vi "ReferenceChannelsToSave.vi"(8 "error in":errorcluster) -> (0 "error out":errorcluster, 1 "Item Names":string[](array[string]), 2 "Value":i32[](array[numeric]), 3 "referenceListBox":refnum<vi>)   [LabVIEW 2016]
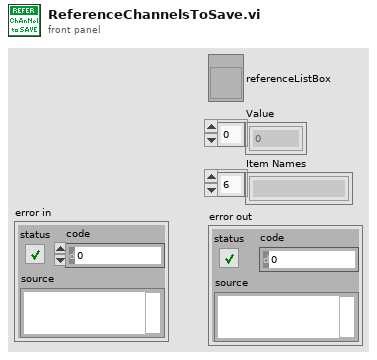
[diagram p1: front panel]
types:
  T1 = enum32{"Invalid", "Standard", "Closed", "Hidden", "Minimized", "Maximized"}
  T2 = enum32{"Bad", "Idle", "Run top level", "Running"}
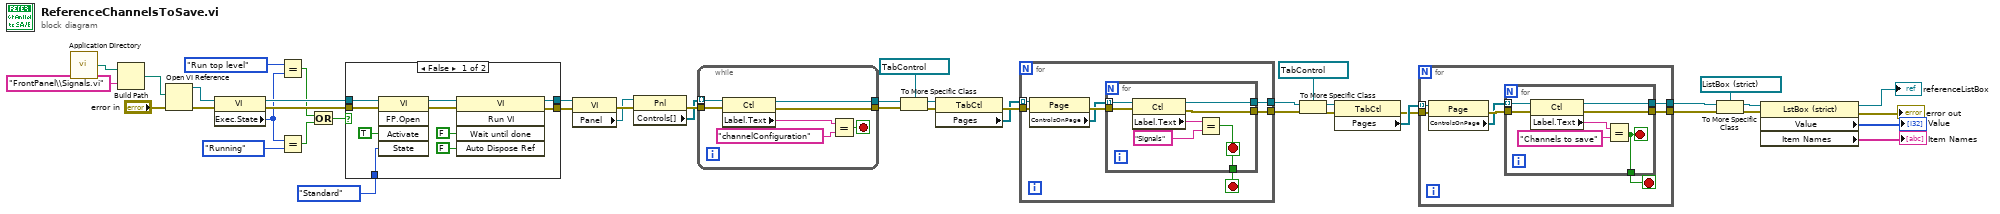
[diagram p0: block diagram]
diagram:
  n1 = call <vilib>:"Application Directory.vi"() -> ("Application Directory"=w38:path)
  n2 = Build Path(base path=w38, name or relative path="FrontPanel\\Signals.vi") -> (appended path=w37:path)
  n3 = Open VI Reference(vi path=w37, error in (no error)="error in") -> (vi reference=w32:refnum<vi>, error out=w30:errorcluster)  [unwired: 4 in]
  n4 = property class="VI"(reference=w32, error in=w30) -> (reference out=w31:refnum<vi>, error out=w29:errorcluster, "Exec.State"=w24:T2)
  n5 = Equal?(x=T2."Run top level" ("Execution:State"), y=w24) -> (x = y?=w26:bool)
  n6 = Equal?(x=w24, y=T2."Running" ("Execution:State")) -> (x = y?=w25:bool)
  n7 = Or(x=w26, y=w25) -> (x .or. y?=w23:bool)
  n8 = case shown="False" w23 {
    tunnel: [w49 w55] -> w34
    tunnel: [w48 w56] -> w33
    tunnel: w31 -> [w47 w56]
    tunnel: w29 -> [w46 w55]
    tunnel: T1."Standard" ("State") -> [w45 _]
    frame False {
      n9 = invoke class="VI" method="FP.Open"(reference=w47, error in=w46, "Activate"=TRUE ("Activate?"), "State"=w45) -> (reference out=w51:refnum<vi>, error out=w50:errorcluster)  [unwired: 1 in, 3 out]
      n10 = invoke class="VI" method="Run VI"(reference=w51, error in=w50, "Wait until done"=FALSE ("Wait Until Done"), "Auto Dispose Ref"=FALSE ("Auto Dispose Reference")) -> (reference out=w48:refnum<vi>, error out=w49:errorcluster)  [unwired: 1 in, 3 out]
    }
    frame True {
    }
  }
  n11 = property class="VI"(reference=w33, error in=w34) -> (error out=w43:errorcluster, "Panel"=w36:refnum<vi>)  [unwired: 1 out]
  n12 = property class="Pnl"(reference=w36, error in=w43) -> (error out=w44:errorcluster, "Controls[]"=w40:refnum<vi>[])  [unwired: 1 out]
  n13 = while {
    tunnel: [w61] -> w41
    tunnel: w40 -> [w60] mode=indexing
    tunnel: w44 -> [w63]
    tunnel: [w62] -> w42
    stop <- w57 stop-if-true
    n14 = property class="Ctl"(reference=w60, error in=w63) -> (reference out=w61:refnum<vi>, error out=w62:errorcluster, "Label.Text"=w58:string)
    n15 = Equal?(x=w58, y="channelConfiguration") -> (x = y?=w57:bool)
  }
  n16 = To More Specific Class(target class=refnum<vi> refnum ("Menus"), reference=w41, error in=w42) -> (specific class reference=w18:refnum<vi>, error out=w21:errorcluster)
  n17 = property class="TabCtl"(reference=w18, error in=w21) -> (error out=w20:errorcluster, "Pages"=w19:refnum<vi>[])  [unwired: 1 out]
  n18 = for {
    tunnel: w19 -> [w69] mode=indexing
    tunnel: [w67] -> w10
    tunnel: [w66] -> w11
    tunnel: w20 -> [w65]
    stop <- w64 stop-if-true
    n19 = property class="Page"(reference=w69, error in=w65) -> (error out=w70:errorcluster, "ControlsOnPage"=w68:refnum<vi>[])  [unwired: 1 out]
    n20 = for {
      tunnel: w68 -> [w77] mode=indexing
      tunnel: [w75] -> w67
      tunnel: [w74] -> w66
      tunnel: w70 -> [w73]
      tunnel: [w71] -> w64
      stop <- w71 stop-if-true
      n21 = property class="Ctl"(reference=w77, error in=w73) -> (reference out=w75:refnum<vi>, error out=w74:errorcluster, "Label.Text"=w72:string)
      n22 = Equal?(x=w72, y="Signals") -> (x = y?=w71:bool)
    }
  }
  n23 = To More Specific Class(target class=refnum<vi> refnum ("Menus"), reference=w10, error in=w11) -> (specific class reference=w15:refnum<vi>, error out=w12:errorcluster)
  n24 = property class="TabCtl"(reference=w15, error in=w12) -> (error out=w13:errorcluster, "Pages"=w14:refnum<vi>[])  [unwired: 1 out]
  n25 = for {
    tunnel: w14 -> [w83] mode=indexing
    tunnel: [w81] -> w9
    tunnel: [w80] -> w8
    tunnel: w13 -> [w79]
    stop <- w78 stop-if-true
    n26 = property class="Page"(reference=w83, error in=w79) -> (error out=w84:errorcluster, "ControlsOnPage"=w82:refnum<vi>[])  [unwired: 1 out]
    n27 = for {
      tunnel: w82 -> [w91] mode=indexing
      tunnel: [w90] -> w81
      tunnel: [w89] -> w80
      tunnel: w84 -> [w88]
      tunnel: [w85] -> w78
      stop <- w85 stop-if-true
      n28 = property class="Ctl"(reference=w91, error in=w88) -> (reference out=w90:refnum<vi>, error out=w89:errorcluster, "Label.Text"=w86:string)
      n29 = Equal?(x=w86, y="Channels to save" ("Label.Text")) -> (x = y?=w85:bool)
    }
  }
  n30 = To More Specific Class(target class=refnum<vi> refnum ("CtlRef"), reference=w9, error in=w8) -> (specific class reference=w7:refnum<vi>, error out=w6:errorcluster)
  n31 = property class="LstBox (strict)"(reference=w7, error in=w6) -> (reference out=→"referenceListBox":refnum<vi>, error out=→"error out":errorcluster, "Value"=→"Value":i32[], "Item Names"=→"Item Names":string[])
